vi "simple_strain_test2.vi"() -> ()   [LabVIEW 2013]
uses:
  ctl/strain_ctl.ctl
  <vilib>/Analysis/baseanly.llb/Mean (DBL).vi
  <vilib>/Analysis/NI_AALBase.lvlib
panel:
  out "XY 그래프 4":cluster{"X":dbl, "Y":dbl}[](graph)
  out "XY 그래프 3":cluster{"X":dbl, "Y":dbl}[](graph)
  in  "정지":bool
  in  "cal":bool
  in  "탭 컨트롤":enum32{"페이지 1", "페이지 2", "페이지 3", "페이지 4"}(tab)
  out "웨이브폼 차트":cluster{dbl, dbl, dbl, dbl}(graph)
  out "XY 그래프 2":cluster{"X":dbl, "Y":dbl}[](graph)
  out "XY 그래프":cluster{"X":dbl, "Y":dbl}[](graph)
  out "예측":cluster{dbl, dbl, dbl, dbl}(graph)
  out "웨이브폼 그래프":waveform(dbl)[](graph)
  out "웨이브폼 그래프 2":waveform(dbl)[](graph)
  out "p 4":dbl
  out "p 3":dbl
  out "p 2":dbl
  out "p 1":dbl
  out "mean 4":dbl caption="평균 f4" format="%.6f"
  out "mean 3":dbl caption="평균 f3" format="%.6f"
  out "mean 2":dbl caption="평균 f2" format="%.6f"
  out "mean 5":dbl caption="평균 f1" format="%.6f"
  out "실측-예측":cluster{dbl, dbl, dbl, dbl}(graph)
  out "숫자형":i32
  out "Strain_offset_data":waveform(dbl)[](array[waveform])
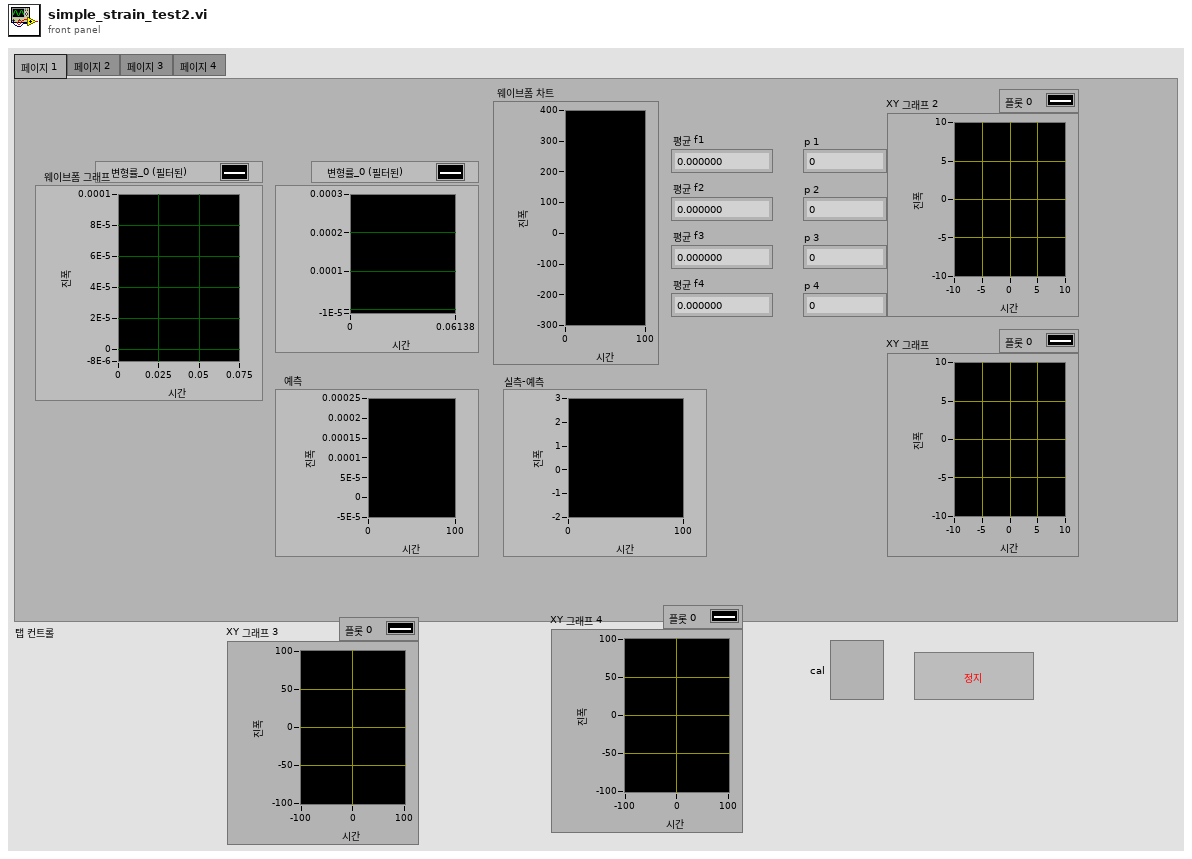
[diagram p1: front panel]
types:
  T1 = typedef "strain_ctl.ctl" = enum16{"config", "start", "read", "close"}
  T2 = cluster{"mean":dbl, "mean":dbl, "mean":dbl, "mean":dbl}[]
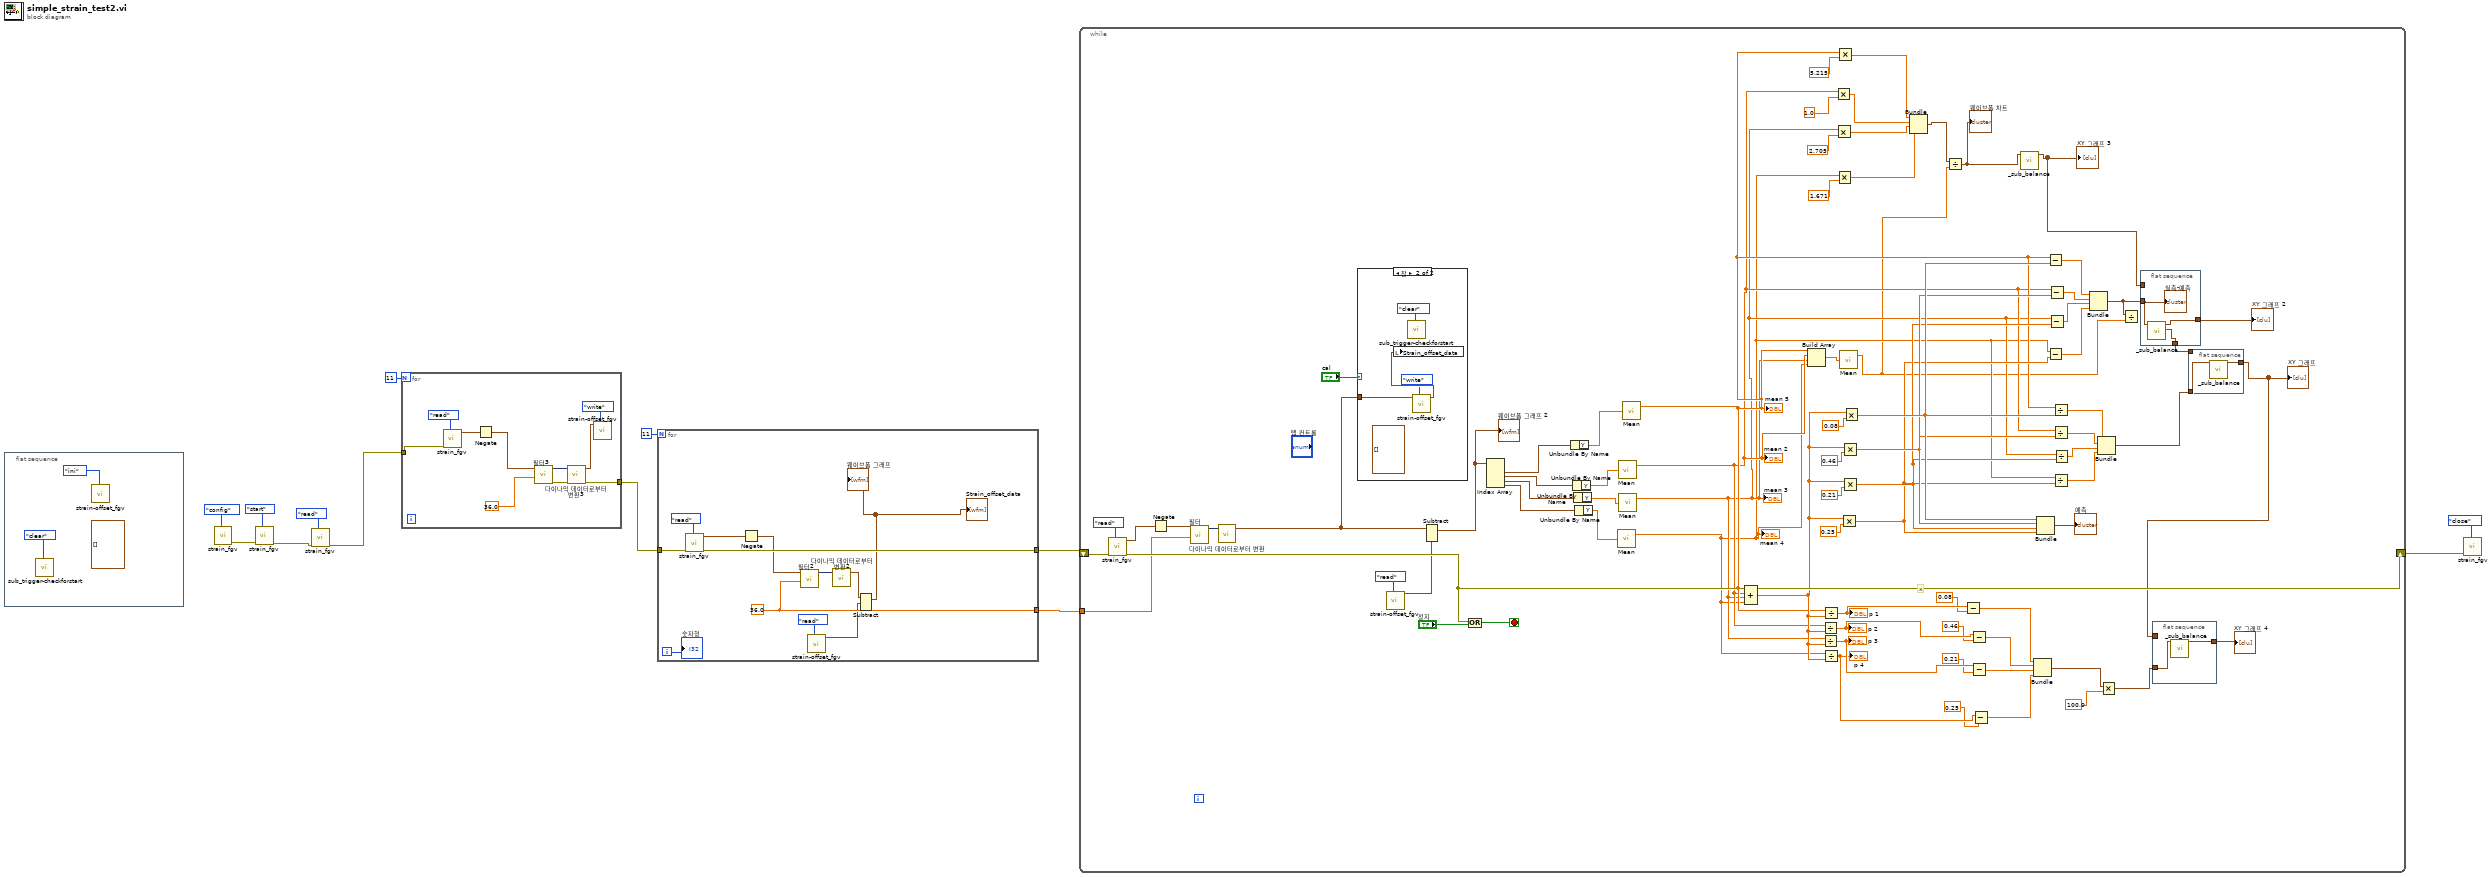
[diagram p0: block diagram]
diagram:
  n1 = flat-sequence {
    frame #0 {
      (unwired) T2 [] ("히스토리 데이터")
      n2 = call "sub_trigger-checkforstart.vi"("check"=enum16{"check", "clear"}."clear") -> ()  [unwired: 7 in, 4 out]
      n3 = call "strain-offset_fgv.vi"("cmd"=enum16{"ini", "write", "read"}."ini") -> ()  [unwired: 10 in, 1 out]
    }
  }
  n4 = call "strain_fgv.vi"("cmd"=strain_ctl."config") -> ("error out"=w9:errorcluster)  [unwired: 9 in, 1 out]
  n5 = call "strain_fgv.vi"("cmd"=strain_ctl."start", "error in"=w9) -> ("error out"=w4:errorcluster)  [unwired: 8 in, 1 out]
  n6 = call "strain_fgv.vi"("cmd"=strain_ctl."read", "error in"=w4) -> ("error out"=w3:errorcluster)  [unwired: 8 in, 1 out]
  n7 = for {
    N: 11 -> [_]
    tunnel: w3 -> [w19]
    tunnel: [w18] -> w2
    n8 = call "strain_fgv.vi"("cmd"=strain_ctl."read", "error in"=w19) -> ("data"=w21:waveform(dbl)[])  [unwired: 8 in, 1 out]
    n9 = Negate(x=w21) -> (-x=w23:waveform(dbl)[])
    n10 = call "필터3"("Lower Cut-Off"=36.0, "Signal"=w23) -> ("error out"=w18:errorcluster, "Filtered Signal"=w20:dynamicdata)  [unwired: 8 in]
    n11 = call "다이나믹 데이터로부터 변환3"("Dynamic Data Type"=w20) -> ("Array of Waveform"=w16:waveform(dbl)[])  [unwired: 3 in]
    n12 = call "strain-offset_fgv.vi"("cmd"=enum16{"ini", "write", "read"}."write", "data"=w16) -> ()  [unwired: 9 in, 1 out]
  }
  n13 = for {
    N: 11 -> [_]
    tunnel: [w36] -> w8
    tunnel: [w33] -> w7
    tunnel: w2 -> [w26]
    i -> [w30]
    w33 = 36.0 ("Lower Cut-Off")
    n14 = call "strain_fgv.vi"("cmd"=strain_ctl."read", "error in"=w26) -> ("error out"=w36:errorcluster, "data"=w34:waveform(dbl)[])  [unwired: 8 in]
    n15 = Negate(x=w34) -> (-x=w32:waveform(dbl)[])
    n16 = call "필터2"("Lower Cut-Off"=w33, "Signal"=w32) -> ("Filtered Signal"=w35:dynamicdata)  [unwired: 8 in, 1 out]
    n17 = call "strain-offset_fgv.vi"("cmd"=enum16{"ini", "write", "read"}."read") -> ("Strain_offset_data"=w27:waveform(dbl)[])  [unwired: 10 in]
    n18 = call "다이나믹 데이터로부터 변환2"("Dynamic Data Type"=w35) -> ("Array of Waveform"=w28:waveform(dbl)[])  [unwired: 3 in]
    n19 = Subtract(1:w27, 2:w28) -> (0:→"Strain_offset_data" →"웨이브폼 그래프":waveform(dbl)[])  [unwired: 1 in, 1 out]
    "숫자형" <- w30
  }
  n20 = while {
    shift-right: [w111] -> w13
    shift-left: w8 -> [w113]
    tunnel: w7 -> [w97]
    stop <- w112 stop-if-true
    # "x"
    n21 = call "strain_fgv.vi"("cmd"=strain_ctl."read", "error in"=w113) -> ("error out"=w111:errorcluster, "data"=w96:waveform(dbl)[])  [unwired: 8 in]
    n22 = Negate(x=w96) -> (-x=w95:waveform(dbl)[])
    n23 = call "필터"("Lower Cut-Off"=w97, "Signal"=w95) -> ("Filtered Signal"=w101:dynamicdata)  [unwired: 8 in, 1 out]
    n24 = call "다이나믹 데이터로부터 변환"("Dynamic Data Type"=w101) -> ("Array of Waveform"=w98:waveform(dbl)[])  [unwired: 3 in]
    n25 = case shown="참" "cal" {
      tunnel: w98 -> [_ w125]
      frame False {
      }
      frame True {
        (unwired) T2 [] ("히스토리 데이터")
        n26 = call "sub_trigger-checkforstart.vi"("check"=enum16{"check", "clear"}."clear") -> ()  [unwired: 7 in, 4 out]
        n27 = call "strain-offset_fgv.vi"("cmd"=enum16{"ini", "write", "read"}."write", "data"=w125) -> ("Strain_offset_data"=w124:waveform(dbl)[])  [unwired: 9 in]
        n28 = local write "Strain_offset_data"(w124) -> ()
      }
    }
    n29 = call "strain-offset_fgv.vi"("cmd"=enum16{"ini", "write", "read"}."read") -> ("Strain_offset_data"=w99:waveform(dbl)[])  [unwired: 10 in]
    n30 = Subtract(1:w99, 2:w98) -> (0:w93:waveform(dbl)[])  [unwired: 1 in, 1 out]
    "웨이브폼 그래프 2" <- w93
    n31 = Compound Arithmetic op=OR(w111, "정지") -> (w112:bool)
    n32 = Index Array(array=w93) -> (element #1=w109:waveform(dbl), element #2=w108:waveform(dbl), element #3=w107:waveform(dbl), element #4=w106:waveform(dbl))  [unwired: 4 in]
    n33 = Unbundle By Name(w109) -> ("Y"=w105:dbl[])
    n34 = Unbundle By Name(w108) -> ("Y"=w102:dbl[])
    n35 = Unbundle By Name(w107) -> ("Y"=w103:dbl[])
    n36 = Unbundle By Name(w106) -> ("Y"=w104:dbl[])
    n37 = call-poly <vilib>:"Mean.vi"("X"=w104) -> ("mean"=w62:dbl)  [unwired: 1 out]
    "mean 4" <- w62
    n38 = call-poly <vilib>:"Mean.vi"("X"=w102) -> ("mean"=w64:dbl)  [unwired: 1 out]
    "mean 2" <- w64
    n39 = call-poly <vilib>:"Mean.vi"("X"=w103) -> ("mean"=w63:dbl)  [unwired: 1 out]
    "mean 3" <- w63
    n40 = call-poly <vilib>:"Mean.vi"("X"=w105) -> ("mean"=w69:dbl)  [unwired: 1 out]
    "mean 5" <- w69
    n41 = Compound Arithmetic op=ADD(w69, w64, w63, w62) -> (w83:dbl)
    n42 = Build Array(w69, w64, w63, w62) -> (w71:dbl[])
    n43 = Divide(x=w64, y=w83) -> (x/y=w45:dbl)
    "p 2" <- w45
    n44 = Divide(x=w63, y=w83) -> (x/y=w43:dbl)
    "p 3" <- w43
    n45 = Divide(x=w69, y=w83) -> (x/y=w47:dbl)
    "p 1" <- w47
    n46 = Divide(x=w62, y=w83) -> (x/y=w41:dbl)
    "p 4" <- w41
    n47 = Multiply(x=w64, y=1.0) -> (x*y=w60:dbl)
    n48 = Multiply(x=w63, y=2.705) -> (x*y=w59:dbl)
    n49 = Multiply(x=w62, y=1.671) -> (x*y=w58:dbl)
    n50 = Multiply(x=w69, y=5.215) -> (x*y=w61:dbl)
    n51 = call-poly <vilib>:"Mean.vi"("X"=w71) -> ("mean"=w57:dbl)  [unwired: 1 out]
    n52 = Multiply(x=w83, y=0.25) -> (x*y=w79:dbl)
    n53 = Multiply(x=w83, y=0.46) -> (x*y=w81:dbl)
    n54 = Multiply(x=w83, y=0.21) -> (x*y=w80:dbl)
    n55 = Multiply(x=w83, y=0.08) -> (x*y=w82:dbl)
    n56 = Bundle(w61, w60, w59, w58) -> (w56:cluster{dbl, dbl, dbl, dbl})  [unwired: 1 in]
    n57 = Divide(x=w56, y=w57) -> (x/y=w55:cluster{dbl, dbl, dbl, dbl})
    "웨이브폼 차트" <- w55
    n58 = Subtract(x=w47, y=0.08) -> (x-y=w53:dbl)
    n59 = Subtract(x=w45, y=0.46) -> (x-y=w52:dbl)
    n60 = Subtract(x=w43, y=0.21) -> (x-y=w51:dbl)
    n61 = Subtract(x=w41, y=0.25) -> (x-y=w50:dbl)
    n62 = call "_sub_balance.vi"("클러스터"=w55) -> ("Balance"=w54:cluster{"X":dbl, "Y":dbl}[])  [unwired: 9 in, 1 out]
    "XY 그래프 3" <- w54
    n63 = Bundle(w53, w52, w51, w50) -> (w39:cluster{dbl, dbl, dbl, dbl})  [unwired: 1 in]
    n64 = Bundle(w82, w81, w80, w79) -> (→"예측":cluster{dbl, dbl, dbl, dbl})  [unwired: 1 in]
    n65 = Subtract(x=w69, y=w82) -> (x-y=w87:dbl)
    n66 = Subtract(x=w62, y=w79) -> (x-y=w84:dbl)
    n67 = Subtract(x=w64, y=w81) -> (x-y=w86:dbl)
    n68 = Subtract(x=w63, y=w80) -> (x-y=w85:dbl)
    n69 = Divide(x=w69, y=w82) -> (x/y=w75:dbl)
    n70 = Divide(x=w64, y=w81) -> (x/y=w76:dbl)
    n71 = Divide(x=w62, y=w79) -> (x/y=w78:dbl)
    n72 = Divide(x=w63, y=w80) -> (x/y=w77:dbl)
    n73 = Bundle(w87, w86, w85, w84) -> (w70:cluster{dbl, dbl, dbl, dbl})  [unwired: 1 in]
    n74 = Bundle(w75, w76, w77, w78) -> (w74:cluster{dbl, dbl, dbl, dbl})  [unwired: 1 in]
    n75 = Multiply(x=w39, y=100.0) -> (x*y=w37:cluster{dbl, dbl, dbl, dbl})
    n76 = Divide(x=w70, y=w57) -> ()  [unwired: 1 out]
    n77 = flat-sequence {
      tunnel: [w119] -> w73
      tunnel: [w118] -> w72
      tunnel: w70 -> [w117]
      tunnel: w54 -> [_]
      frame #0 {
        n78 = call "_sub_balance.vi"("클러스터"=w117) -> ("Balance xy wfs"=w119:cluster{"X":dbl, "Y":dbl}[], "Balance"=w118:cluster{"X":dbl, "Y":dbl}[])  [unwired: 9 in]
        "실측-예측" <- w117
      }
    }
    n79 = flat-sequence {
      tunnel: w37 -> [w116]
      tunnel: w49 -> [_]
      tunnel: [w115] -> w48
      frame #0 {
        n80 = call "_sub_balance.vi"("클러스터"=w116) -> ("Balance"=w115:cluster{"X":dbl, "Y":dbl}[])  [unwired: 9 in, 1 out]
      }
    }
    n81 = flat-sequence {
      tunnel: [w121] -> w49
      tunnel: w74 -> [w120]
      tunnel: w73 -> [_]
      frame #0 {
        n82 = call "_sub_balance.vi"("클러스터"=w120) -> ("Balance"=w121:cluster{"X":dbl, "Y":dbl}[])  [unwired: 9 in, 1 out]
      }
    }
    "XY 그래프" <- w49
    "XY 그래프 2" <- w72
    "XY 그래프 4" <- w48
  }
  n83 = call "strain_fgv.vi"("cmd"=strain_ctl."close", "error in"=w13) -> ()  [unwired: 8 in, 2 out]
